vi "Remove Close Atoms.vi"(9 "Edge Duplication Range":dbl=3.0, 10 "Minimally Allowable Distance (A)":dbl=1.5, 11 "Structure":T1={"Structure Name"="Relax2 Subcrystal Expanded to Box+Relax2 Subcrystal Expanded to Box", "Lattice vector a"=[10.1, 0.0, 0.0], "Lattice vector b"=[0.0, 100.1, 0.0], "Lattice vector c"=[0.0, 0.0, 24.72380952380952], "Atoms Array"=[{"Atom Name"="Cd", "Positions (Direct)"=array496x3[1488 elements], "Positions (Cartesian)"=array496x3[1488 elements]}, {"Atom Name"="Te", "Positions (Direct)"=array480x3[1440 elements], "Positions (Cartesian)"=array480x3[1440 elements]}], "# of atoms"=976} {"Atoms Array"."Positions (Cartesian)" format="%#_4f"; "Atoms Array"."Positions (Direct)" format="%#_4f"}) -> (2 "# of Atoms Removed":i32, 3 "Structure with atoms removed":T1={"Structure Name"="Relax2 Subcrystal Expanded to Box+Relax2 Subcrystal Expanded to Box", "Lattice vector a"=[10.1, 0.0, 0.0], "Lattice vector b"=[0.0, 100.1, 0.0], "Lattice vector c"=[0.0, 0.0, 24.72380952380952], "Atoms Array"=[{"Atom Name"="Cd", "Positions (Direct)"=array496x3[1488 elements], "Positions (Cartesian)"=array496x3[1488 elements]}, {"Atom Name"="Te", "Positions (Direct)"=array480x3[1440 elements], "Positions (Cartesian)"=array480x3[1440 elements]}], "# of atoms"=976} {"Atoms Array"."Positions (Cartesian)" format="%#_4f"; "Atoms Array"."Positions (Direct)" format="%#_4f"})   [LabVIEW 2010]
uses:
  <vilib>/Analysis/_algsub.llb/Real Vector Norm.vi
  <vilib>/Analysis/NI_AALPro.lvlib
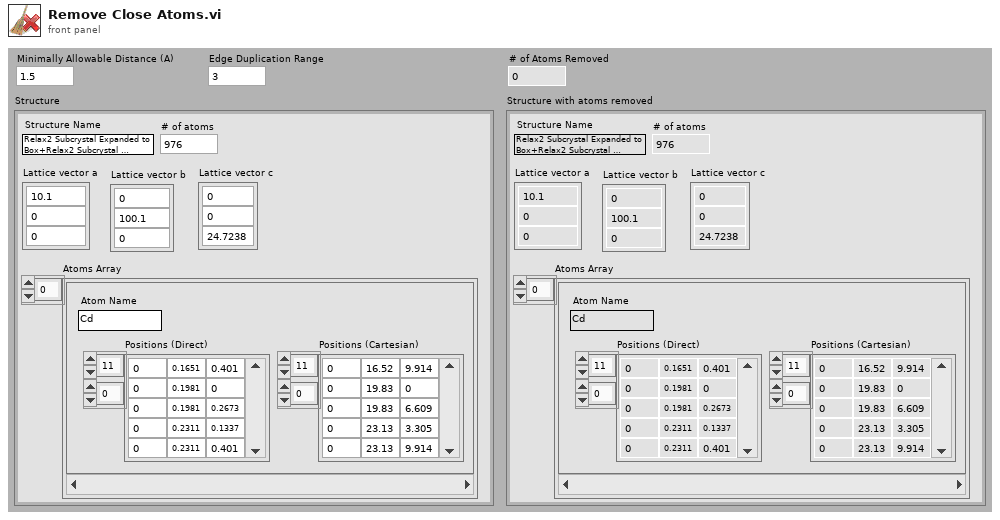
[diagram p1: front panel]
types:
  T1 = cluster{"Structure Name":string, "Lattice vector a":dbl[], "Lattice vector b":dbl[], "Lattice vector c":dbl[], "Atoms Array":cluster{"Atom Name":string, "Positions (Direct)":dbl[][], "Positions (Cartesian)":dbl[][]}[], "# of atoms":i32}
  T2 = cluster{"Atom Name":string, "Positions (Direct)":dbl[][], "Positions (Cartesian)":dbl[][]}[]
  T3 = cluster{"Atom Name":string, "Positions (Direct)":dbl[][], "Positions (Cartesian)":dbl[][]}
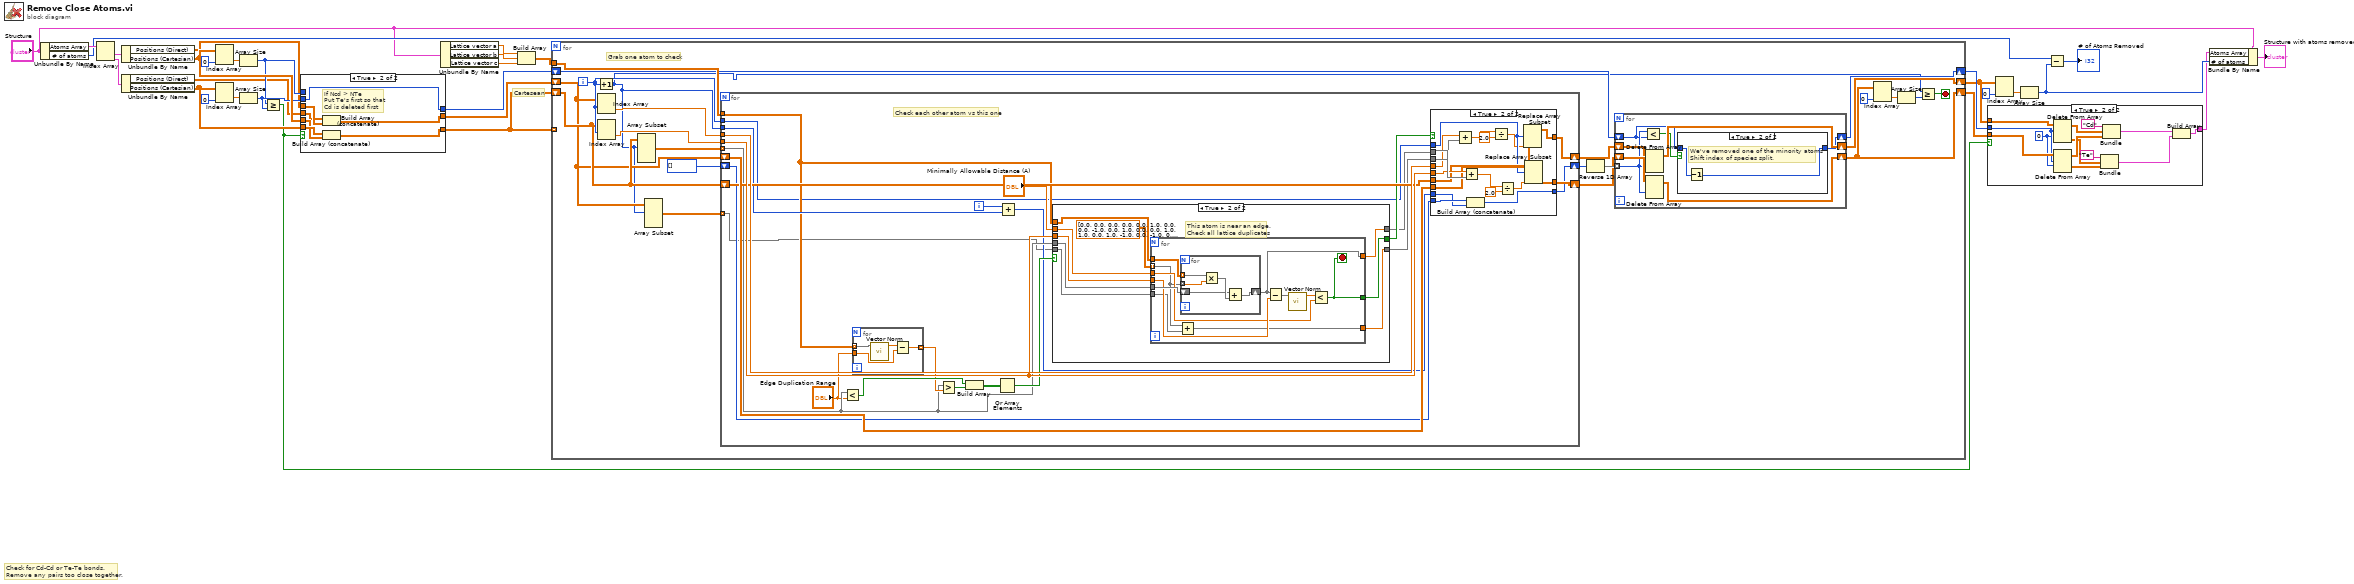
[diagram p0: block diagram]
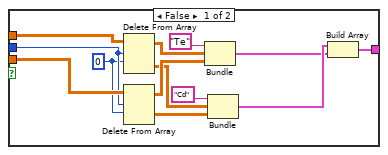
[diagram p2: hidden frame]
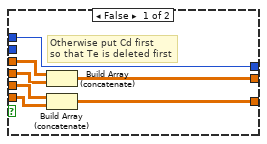
[diagram p3: hidden frame]
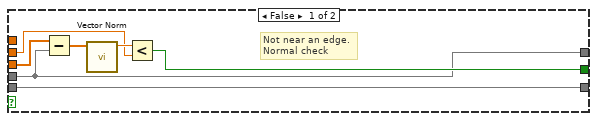
[diagram p5: hidden frame]
diagram:
  # "Cartesean"
  # "Check for Cd-Cd or Te-Te bonds.\nRemove any pairs too close together."
  n1 = Unbundle By Name("Structure") -> ("Atoms Array"=w31:T2, "# of atoms"=w9:i32)
  n2 = Index Array(array=w31) -> (element #1=w30:T3, element #2=w29:T3)  [unwired: 2 in]
  n3 = Unbundle By Name(w30) -> ("Positions (Direct)"=w16:dbl[][], "Positions (Cartesian)"=w24:dbl[][])
  n4 = Unbundle By Name(w29) -> ("Positions (Direct)"=w15:dbl[][], "Positions (Cartesian)"=w23:dbl[][])
  n5 = Index Array(array=w24, index (col)=0 ("disabled index (col)")) -> (element=w27:dbl[])  [unwired: 1 in]
  n6 = Index Array(array=w23, index (col)=0 ("disabled index (col)")) -> (element=w25:dbl[])  [unwired: 1 in]
  n7 = Array Size(array=w27) -> (size(s)=w19:i32)
  n8 = Array Size(array=w25) -> (size(s)=w20:i32)
  n9 = Greater Or Equal?(x=w19, y=w20) -> (x >= y?=w21:bool)
  n10 = case shown="True" w21 {
    tunnel: w24 -> [w39 w45]
    tunnel: [w38 w44] -> w3
    tunnel: w23 -> [w37 w46]
    tunnel: [w36 w43] -> w18
    tunnel: w20 -> [_ w43]
    tunnel: w19 -> [w36 _]
    tunnel: w16 -> [w35 w42]
    tunnel: w15 -> [w34 w41]
    tunnel: [w33 w40] -> w14
    frame False {
      # "Otherwise put Cd first\nso that Te is deleted first"
      n11 = Build Array (concatenate)(w35, w34) -> (w33:dbl[][])
      n12 = Build Array (concatenate)(w39, w37) -> (w38:dbl[][])
    }
    frame True {
      # "If Ncd > NTe\nPut Te's first so that\nCd is deleted first"
      n13 = Build Array (concatenate)(w41, w42) -> (w40:dbl[][])
      n14 = Build Array (concatenate)(w46, w45) -> (w44:dbl[][])
    }
  }
  n15 = Unbundle By Name("Structure") -> ("Lattice vector a"=w6:dbl[], "Lattice vector b"=w7:dbl[], "Lattice vector c"=w5:dbl[])
  n16 = Build Array(w6, w7, w5) -> (w4:dbl[][])
  n17 = for {
    shift-right: [w53] -> w22
    shift-left: w3 -> [w60]
    shift-right: [w50] -> w17
    shift-left: w18 -> [w51]
    shift-right: [w52] -> w13
    shift-left: w14 -> [w49]
    tunnel: w4 -> [w58]
    tunnel: w3 -> [_] mode=indexing
    i -> [w61]
    stop <- w65 stop-if-true
    # "Grab one atom to check"
    n18 = Increment(x=w61) -> (x+1=w48:i32)
    n19 = Index Array(array=w49, index (row)=w61) -> (element=w64:dbl[])  [unwired: 1 in]
    n20 = Index Array(array=w60, index (row)=w61) -> (element=w63:dbl[])  [unwired: 1 in]
    n21 = Array Subset(array=w60, index (row)=w48) -> (w59:dbl[][])  [unwired: 3 in]
    n22 = Array Subset(array=w49, index (row)=w48) -> (w47:dbl[][])  [unwired: 3 in]
    n23 = for {
      tunnel: w63 -> [w102]
      shift-right: [w104] -> w54
      shift-left: w60 -> [w99]
      tunnel: w61 -> [w81]
      shift-right: [w101] -> w55
      shift-left: w49 -> [w100]
      tunnel: w64 -> [w103]
      shift-right: [w97] -> w57
      shift-left: i32[] [] -> [w96]
      tunnel: w59 -> [w86] mode=indexing
      tunnel: w48 -> [w91]
      tunnel: w58 -> [w83]
      tunnel: w47 -> [w80] mode=indexing
      i -> [w92]
      # "Check each other atom vs this one"
      n24 = Less?(x=w86, y="Edge Duplication Range") -> (x < y?=w89:bool[])
      n25 = for {
        tunnel: w83 -> [w108] mode=indexing
        tunnel: "Edge Duplication Range" -> [w106]
        tunnel: [w105] -> w87 mode=indexing
        n26 = call-poly <vilib>:"Vector Norm.vi"("Input Vector"=w108) -> ("norm"=w107:dbl)  [unwired: 9 in, 1 out]
        n27 = Subtract(x=w107, y=w106) -> (x-y=w105:dbl)
      }
      n28 = Greater?(x=w86, y=w87) -> (0:w85:bool[])
      n29 = Build Array(w89, w85) -> (w88:bool[][])
      n30 = Or Array Elements(Boolean array=w88) -> (logical OR=w90:bool)
      n31 = Add(x=w92, y=w91) -> (x+y=w82:i32)
      n32 = case shown="True" w90 {
        tunnel: w86 -> [w110 w122]
        tunnel: "Minimally Allowable Distance (A)" -> [w112 w121]
        tunnel: w102 -> [w115 w123]
        tunnel: [w111 w120] -> w98
        tunnel: [w110 w117] -> w94
        tunnel: w80 -> [w109 w119]
        tunnel: [w109 w118] -> w93
        tunnel: w83 -> [_ w116]
        frame False {
          # "Not near an edge.\nNormal check"
          n33 = Subtract(x=w115, y=w110) -> (x-y=w114:dbl[])
          n34 = call-poly <vilib>:"Vector Norm.vi"("Input Vector"=w114) -> ("norm"=w113:dbl)  [unwired: 9 in, 1 out]
          n35 = Less?(x=w113, y=w112) -> (x < y?=w111:bool)
        }
        frame True {
          # "This atom is near an edge.\nCheck all lattice duplicates"
          n36 = for {
            tunnel: w122 -> [w135]
            tunnel: dbl[][] [[0.0, 0.0, 0.0], [0.0, 0.0, 1.0], [0.0, 0.0, -1.0], [0.0, 1.0, 0.0], [0.0, 1.0, 1.0], [0.0, 1.0, -1.0], [0.0, -1.0, 0.0], [0.0, -1.0, 1.0], [0.0, -1.0, -1.0], [1.0, 0.0, 0.0], [1.0, 0.0, 1.0], [1.0, 0.0, -1.0], [1.0, 1.0, 0.0], [1.0, 1.0, 1.0], [1.0, 1.0, -1.0], [1.0, -1.0, 0.0], [1.0, -1.0, 1.0], [1.0, -1.0, -1.0], [-1.0, 0.0, 0.0], [-1.0, 0.0, 1.0], [-1.0, 0.0, -1.0], [-1.0, 1.0, 0.0], [-1.0, 1.0, 1.0], [-1.0, 1.0, -1.0], [-1.0, -1.0, 0.0], [-1.0, -1.0, 1.0], [-1.0, -1.0, -1.0]] ("Array") -> [w125] mode=indexing
            tunnel: [w126] -> w117
            tunnel: w116 -> [w134]
            tunnel: w123 -> [w133]
            tunnel: w121 -> [w130]
            tunnel: [w129] -> w120
            tunnel: [w128] -> w118
            tunnel: w119 -> [w127]
            stop <- w129 stop-if-true
            n37 = Add(x=w125, y=w127) -> (x+y=w128:dbl[])
            n38 = for {
              shift-right: [w136] -> w126
              shift-left: w135 -> [w137]
              tunnel: w125 -> [w140] mode=indexing
              tunnel: w134 -> [w139] mode=indexing
              n39 = Multiply(x=w139, y=w140) -> (x*y=w138:dbl[])
              n40 = Add(x=w137, y=w138) -> (x+y=w136:dbl[])
            }
            n41 = Subtract(x=w126, y=w133) -> (x-y=w132:dbl[])
            n42 = call-poly <vilib>:"Vector Norm.vi"("Input Vector"=w132) -> ("norm"=w131:dbl)  [unwired: 9 in, 1 out]
            n43 = Less?(x=w131, y=w130) -> (x < y?=w129:bool)
          }
        }
      }
      n44 = case shown="True" w98 {
        tunnel: w99 -> [w143 w157]
        tunnel: [w143 w147] -> w104
        tunnel: w81 -> [_ w153]
        tunnel: w94 -> [_ w159]
        tunnel: w102 -> [_ w158]
        tunnel: w100 -> [w142 w154]
        tunnel: [w142 w148] -> w101
        tunnel: w93 -> [_ w151]
        tunnel: w103 -> [_ w150]
        tunnel: [w141 w146] -> w97
        tunnel: w96 -> [w141 w145]
        tunnel: w82 -> [_ w144]
        frame False {
        }
        frame True {
          n45 = Add(x=w150, y=w151) -> (x+y=w152:dbl[])
          n46 = Add(x=w158, y=w159) -> (x+y=w160:dbl[])
          n47 = Build Array (concatenate)(w145, w144) -> (w146:i32[])
          n48 = Divide(x=w152, y=2.0) -> (x/y=w149:dbl[])
          n49 = Divide(x=w160, y=2.0) -> (x/y=w156:dbl[])
          n50 = Replace Array Subset(array=w154, new element=w149, index (row)=w153) -> (w148:dbl[][])  [unwired: 1 in]
          n51 = Replace Array Subset(array=w157, new element=w156, index (row)=w153) -> (w147:dbl[][])  [unwired: 1 in]
        }
      }
    }
    n52 = Reverse 1D Array(array=w57) -> (reversed array=w56:i32[])
    n53 = for {
      shift-right: [w75] -> w52
      shift-left: w55 -> [w76]
      tunnel: w56 -> [w71] mode=indexing
      shift-right: [w73] -> w53
      shift-left: w54 -> [w74]
      shift-right: [w72] -> w50
      shift-left: w51 -> [w70]
      n54 = Less?(x=w71, y=w70) -> (x < y?=w69:bool)
      n55 = Delete From Array(array=w76, index (row)=w71) -> (array with subset deleted=w75:dbl[][])  [unwired: 2 in, 1 out]
      n56 = Delete From Array(array=w74, index (row)=w71) -> (array with subset deleted=w73:dbl[][])  [unwired: 2 in, 1 out]
      n57 = case shown="True" w69 {
        tunnel: [w77 w79] -> w72
        tunnel: w70 -> [w77 w78]
        frame False {
        }
        frame True {
          # "We've removed one of the minority atoms\nShift index of species split."
          n58 = Decrement(x=w78) -> (x-1=w79:i32)
        }
      }
    }
    n59 = Index Array(array=w53, index (col)=0 ("disabled index (col)")) -> (element=w67:dbl[])  [unwired: 1 in]
    n60 = Array Size(array=w67) -> (size(s)=w66:i32)
    n61 = Greater Or Equal?(x=w48, y=w66) -> (x >= y?=w65:bool)
  }
  n62 = case shown="True" w21 {
    tunnel: w22 -> [w174 w187]
    tunnel: [w169 w184] -> w2
    tunnel: w17 -> [w165 w178]
    tunnel: w13 -> [w166 w179]
    frame False {
      w164 = 0 ("index (row)")
      n63 = Delete From Array(array=w166, length=w165, index (row)=w164) -> (deleted portion=w163:dbl[][], array with subset deleted=w162:dbl[][])  [unwired: 1 in]
      n64 = Delete From Array(array=w174, length=w165, index (row)=w164) -> (deleted portion=w168:dbl[][], array with subset deleted=w167:dbl[][])  [unwired: 1 in]
      n65 = Bundle("Te", w162, w167) -> (w170:cluster{string, dbl[][], dbl[][]})  [unwired: 1 in]
      n66 = Bundle("Cd", w163, w168) -> (w172:cluster{string, dbl[][], dbl[][]})  [unwired: 1 in]
      n67 = Build Array(w172, w170) -> (w169:cluster{string, dbl[][], dbl[][]}[])
    }
    frame True {
      w177 = 0 ("index (row)")
      n68 = Delete From Array(array=w179, length=w178, index (row)=w177) -> (deleted portion=w175:dbl[][], array with subset deleted=w176:dbl[][])  [unwired: 1 in]
      n69 = Delete From Array(array=w187, length=w178, index (row)=w177) -> (deleted portion=w181:dbl[][], array with subset deleted=w180:dbl[][])  [unwired: 1 in]
      n70 = Bundle("Te", w175, w181) -> (w182:cluster{string, dbl[][], dbl[][]})  [unwired: 1 in]
      n71 = Bundle("Cd", w176, w180) -> (w185:cluster{string, dbl[][], dbl[][]})  [unwired: 1 in]
      n72 = Build Array(w185, w182) -> (w184:cluster{string, dbl[][], dbl[][]}[])
    }
  }
  n73 = Index Array(array=w13, index (col)=0 ("disabled index (col)")) -> (element=w11:dbl[])  [unwired: 1 in]
  n74 = Array Size(array=w11) -> (size(s)=w10:i32)
  n75 = Subtract(x=w9, y=w10) -> (x-y=→"# of Atoms Removed":i32)
  n76 = Bundle By Name(cluster="Structure", "Atoms Array"=w2, "# of atoms"=w10) -> (→"Structure with atoms removed":T1)
